vi "RangeI2C-single_v2.vi"(0 "Remote IP Address":string="192.168.124.53", 1 "Remote Port":u16=502, 2 "I2C Operation Control":T1(ring)=enum."Command Find Range", 3 "SCL DIO Ch. No.":u16=2, 4 "SDA DIO Ch. No.":u16=3, 5 "CURRENT 8-bit address (dec.)":u16=224, 8 "NEW 8-bit address (dec.)":u8=224) -> (6 "Range (cm)":dbl=101.0, 7 "Range (in.)":dbl=39.76377952755905)   [LabVIEW 2014]
panel:
  in  "stop":bool
  # "Even address values up to 254\n\nInvalid Address Values: 0, 80, 164, 170"
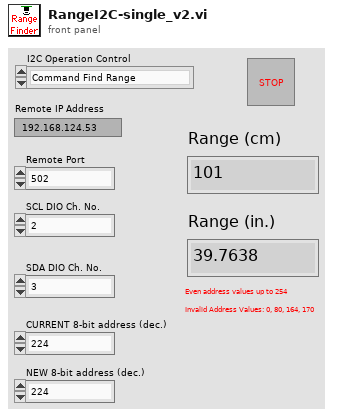
[diagram p1: front panel]
types:
  T1 = enum16{"Configure I2C Settings", "Command Find Range", "Command Read Range", "Report the last range value", "Change sensor address", "Wait to range 100ms"}
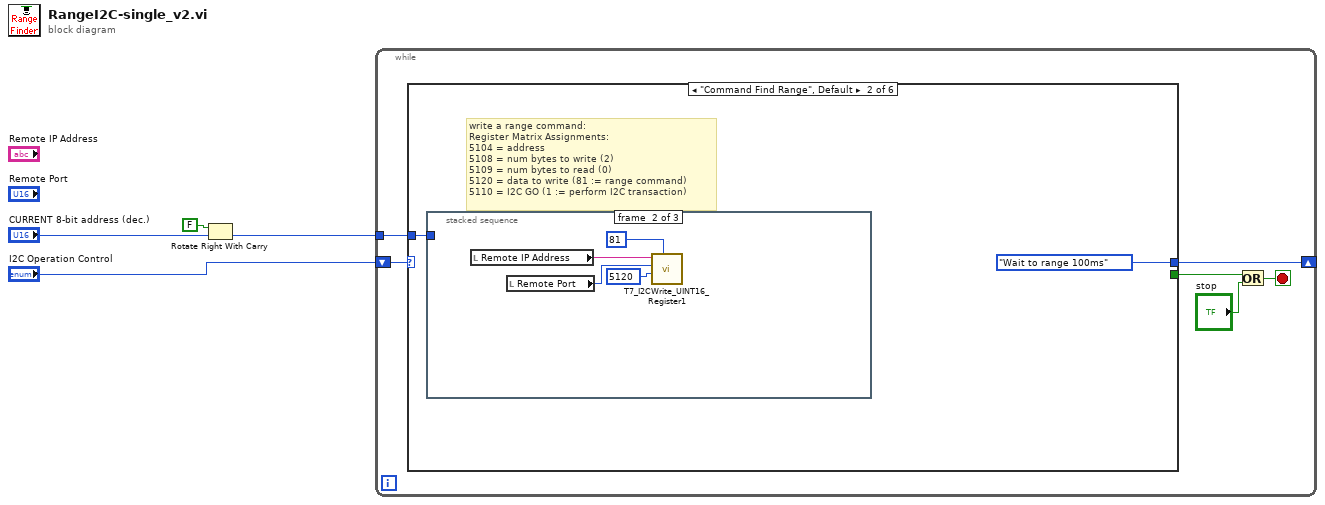
[diagram p0: block diagram]
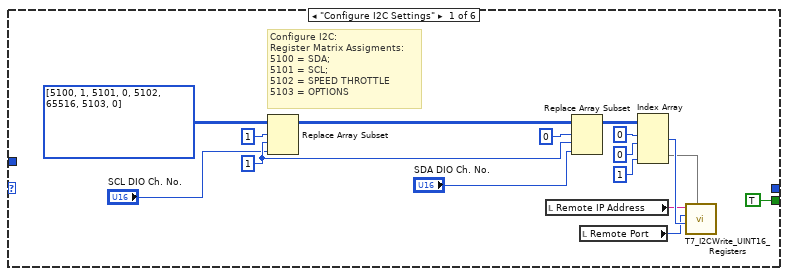
[diagram p2: hidden frame]
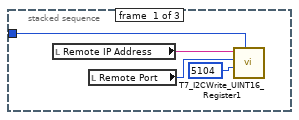
[diagram p3: hidden frame]
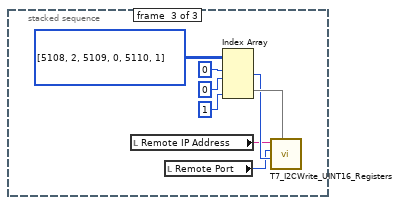
[diagram p4: hidden frame]
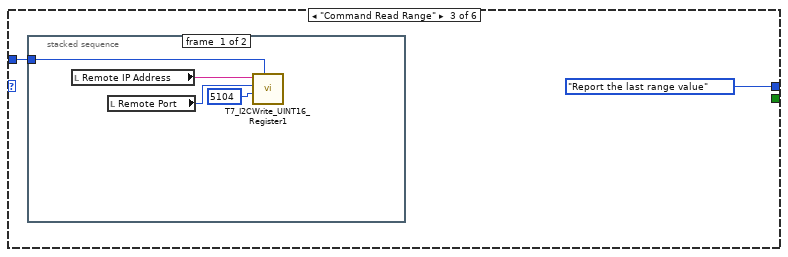
[diagram p5: hidden frame]
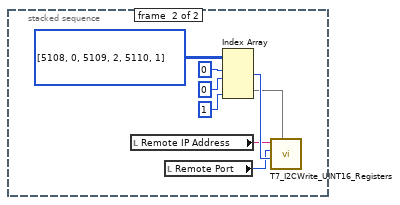
[diagram p6: hidden frame]
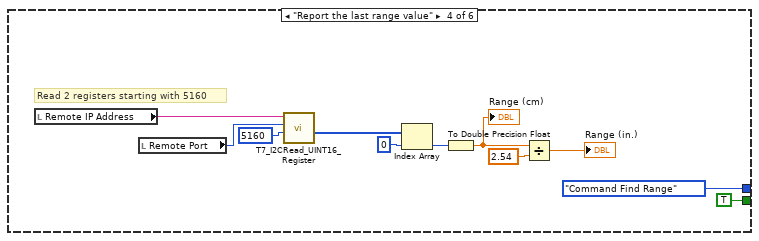
[diagram p7: hidden frame]
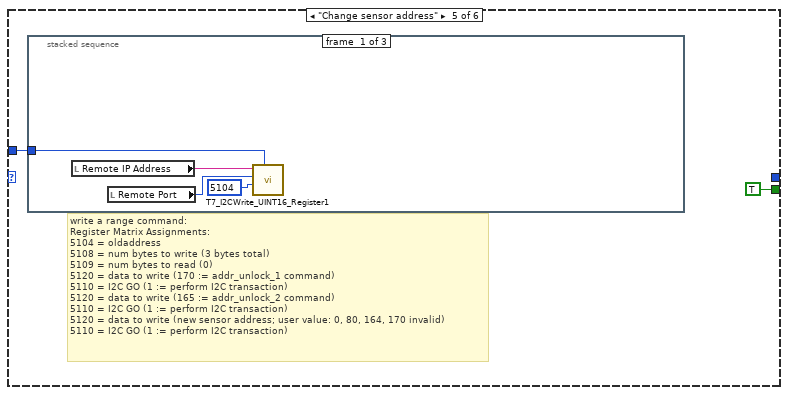
[diagram p8: hidden frame]
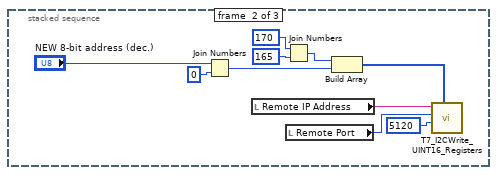
[diagram p9: hidden frame]
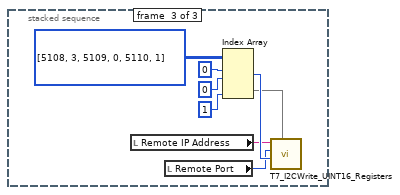
[diagram p10: hidden frame]
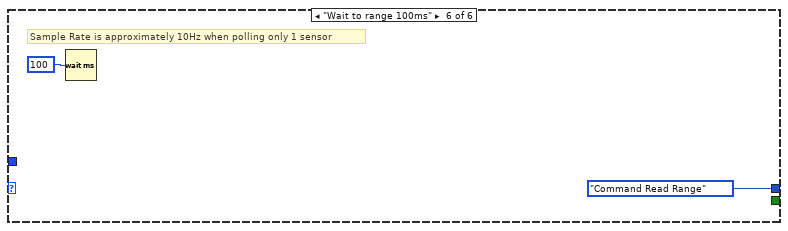
[diagram p11: hidden frame]
diagram:
  n1 = Rotate Right With Carry(2:"CURRENT 8-bit address (dec.)", 3:FALSE ("carry")) -> (0:w1:u16)  [unwired: 1 out]
  n2 = while {
    tunnel: w1 -> [w10]
    shift-right: [w9] -> _
    shift-left: "I2C Operation Control" -> [w5]
    stop <- w6 stop-if-true
    n3 = case shown="\"Command Find Range\", Default" w5 {
      tunnel: w10 -> [_ w27 w45 _ w70 _]
      tunnel: [_ T1."Wait to range 100ms" ("I2C Operation Control") T1."Report the last range value" ("I2C Operation Control") T1."Command Find Range" ("I2C Operation Control") _ T1."Command Read Range" ("I2C Operation Control")] -> w9
      tunnel: [TRUE ("x") _ _ TRUE ("x") TRUE ("x") _] -> w7
      frame "Configure I2C Settings" {
        w21 = 1 ("disabled index (col)")
        # "Configure I2C: \nRegister Matrix Assigments:\n5100 = SDA;\n5101 = SCL;\n5102 = SPEED THROTTLE\n5103 = OPTIONS"
        n4 = Replace Array Subset(array=i32[][] [[5100, 1], [5101, 0], [5102, 65516], [5103, 0]], new element="SCL DIO Ch. No.", index (row)=1, index (col)=w21) -> (w20:i32[][])
        n5 = local read "Remote IP Address"() -> (w12:string)
        n6 = Replace Array Subset(array=w20, new element="SDA DIO Ch. No.", index (row)=0, index (col)=w21) -> (w17:i32[][])
        n7 = local read "Remote Port"() -> (w11:u16)
        n8 = Index Array(array=w17, index (row) #1=0 ("disabled index (row)"), index (col) #1=0 ("disabled index (col)"), index (col) #2=1 ("index (col)")) -> (element #1=w14:i32, element #2=w13:i32[])  [unwired: 1 in]
        n9 = call "T7_I2CWrite_UINT16_Registers.vi"("Remote IP Address"=w12, "Remote Port"=w11, "Starting Address"=w14, "UINT16 to Write"=w13) -> ()  [unwired: 5 in, 2 out]
      }
      frame "Command Find Range", Default {
        # "write a range command:\nRegister Matrix Assignments:\n5104 = address\n5108 = num bytes to write (2)\n5109 = num bytes to read (0)\n5120 = data to write (81 := range command)\n5110 = I2C GO (1 := perform I2C transaction)"
        n10 = stacked-sequence {
          tunnel: w27 -> [w31 _ _]
          frame #0 {
            n11 = local read "Remote IP Address"() -> (w30:string)
            n12 = local read "Remote Port"() -> (w29:u16)
            n13 = call "T7_I2CWrite_UINT16_Register1.vi"("Remote IP Address"=w30, "Remote Port"=w29, "Starting Address"=u16 5104, "UINT16 to Write"=w31) -> ()  [unwired: 5 in, 2 out]
          }
          frame #1 {
            n14 = local read "Remote IP Address"() -> (w34:string)
            n15 = local read "Remote Port"() -> (w33:u16)
            n16 = call "T7_I2CWrite_UINT16_Register1.vi"("Remote IP Address"=w34, "Remote Port"=w33, "Starting Address"=u16 5120, "UINT16 to Write"=81) -> ()  [unwired: 5 in, 2 out]
          }
          frame #2 {
            n17 = local read "Remote IP Address"() -> (w38:string)
            n18 = local read "Remote Port"() -> (w37:u16)
            n19 = Index Array(array=i32[][] [[5108, 2], [5109, 0], [5110, 1]], index (row) #1=0 ("disabled index (row)"), index (col) #1=0 ("disabled index (col)"), index (col) #2=1 ("index (col)")) -> (element #1=w39:i32, element #2=w40:i32[])  [unwired: 1 in]
            n20 = call "T7_I2CWrite_UINT16_Registers.vi"("Remote IP Address"=w38, "Remote Port"=w37, "Starting Address"=w39, "UINT16 to Write"=w40) -> ()  [unwired: 5 in, 2 out]
          }
        }
      }
      frame "Command Read Range" {
        n21 = stacked-sequence {
          tunnel: w45 -> [w49 _]
          frame #0 {
            n22 = local read "Remote IP Address"() -> (w48:string)
            n23 = local read "Remote Port"() -> (w47:u16)
            n24 = call "T7_I2CWrite_UINT16_Register1.vi"("Remote IP Address"=w48, "Remote Port"=w47, "Starting Address"=u16 5104, "UINT16 to Write"=w49) -> ()  [unwired: 5 in, 2 out]
          }
          frame #1 {
            n25 = local read "Remote IP Address"() -> (w52:string)
            n26 = local read "Remote Port"() -> (w51:u16)
            n27 = Index Array(array=i32[][] [[5108, 0], [5109, 2], [5110, 1]], index (row) #1=0 ("disabled index (row)"), index (col) #1=0 ("disabled index (col)"), index (col) #2=1 ("index (col)")) -> (element #1=w54:i32, element #2=w53:i32[])  [unwired: 1 in]
            n28 = call "T7_I2CWrite_UINT16_Registers.vi"("Remote IP Address"=w52, "Remote Port"=w51, "Starting Address"=w54, "UINT16 to Write"=w53) -> ()  [unwired: 5 in, 2 out]
          }
        }
      }
      frame "Report the last range value" {
        # "Read 2 registers starting with 5160"
        n29 = local read "Remote IP Address"() -> (w67:string)
        n30 = local read "Remote Port"() -> (w68:u16)
        n31 = call "T7_I2CRead_UINT16_Register.vi"("FirstChannel"=5160, "Remote Port"=w68, "Remote IP Address"=w67) -> ("Raw Data Read"=w66:u16[])  [unwired: 6 in, 2 out]
        n32 = Index Array(array=w66, index=0) -> (element=w64:u16)
        n33 = To Double Precision Float(number=w64) -> (double precision float=w60:dbl)
        "Range (cm)" <- w60
        n34 = Divide(x=w60, y=2.54) -> (x/y=→"Range (in.)":dbl)
      }
      frame "Change sensor address" {
        # "write a range command:\nRegister Matrix Assignments:\n5104 = oldaddress\n5108 = num bytes to write (3 bytes total)\n5109 = num bytes to read (0)\n5120 = data to write (170 := addr_unlock_1 command)\n5110 = I2C GO (1 := perform I2C transaction)\n5120 = data to write (165 := addr_unlock_2 command)\n5110 = I2C GO (1 := perform I2C transaction)\n5120 = data to write (new sensor address; user value: 0, 80, 164, 170 invalid)\n5110 = I2C GO (1 := perform I2C transaction)"
        n35 = stacked-sequence {
          tunnel: w70 -> [w75 _ _]
          frame #0 {
            n36 = local read "Remote IP Address"() -> (w73:string)
            n37 = local read "Remote Port"() -> (w72:u16)
            n38 = call "T7_I2CWrite_UINT16_Register1.vi"("Remote IP Address"=w73, "Remote Port"=w72, "Starting Address"=u16 5104, "UINT16 to Write"=w75) -> ()  [unwired: 5 in, 2 out]
          }
          frame #1 {
            n39 = Join Numbers(hi="NEW 8-bit address (dec.)", lo=u8 0) -> ((hi.lo)=w81:u16)
            n40 = local read "Remote IP Address"() -> (w83:string)
            n41 = Join Numbers(hi=u8 170, lo=u8 165) -> ((hi.lo)=w80:u16)
            n42 = local read "Remote Port"() -> (w84:u16)
            n43 = Build Array(w80, w81) -> (w82:u16[])
            n44 = call "T7_I2CWrite_UINT16_Registers.vi"("Remote IP Address"=w83, "Remote Port"=w84, "Starting Address"=u16 5120, "UINT16 to Write"=w82) -> ()  [unwired: 5 in, 2 out]
          }
          frame #2 {
            n45 = local read "Remote IP Address"() -> (w87:string)
            n46 = local read "Remote Port"() -> (w86:u16)
            n47 = Index Array(array=i32[][] [[5108, 3], [5109, 0], [5110, 1]], index (row) #1=0 ("disabled index (row)"), index (col) #1=0 ("disabled index (col)"), index (col) #2=1 ("index (col)")) -> (element #1=w89:i32, element #2=w88:i32[])  [unwired: 1 in]
            n48 = call "T7_I2CWrite_UINT16_Registers.vi"("Remote IP Address"=w87, "Remote Port"=w86, "Starting Address"=w89, "UINT16 to Write"=w88) -> ()  [unwired: 5 in, 2 out]
          }
        }
      }
      frame "Wait to range 100ms" {
        # "Sample Rate is approximately 10Hz when polling only 1 sensor"
        n49 = Wait (ms)(milliseconds to wait=u32 100) -> ()  [unwired: 1 out]
      }
    }
    n50 = Or(x=w7, y="stop") -> (x .or. y?=w6:bool)
  }
